vi "ParseRulesFile.vi"(8 "error in (no error)":errorcluster, 9 "Parameters":string, 11 "IRuleFileParser in":refnum<class "IRuleFileParser.lvclass">) -> (0 "error out":errorcluster, 2 "Rules":T1, 3 "IRuleFileParser out":refnum<class "IRuleFileParser.lvclass">)   [LabVIEW 2020, in "ExtensionInterfaces.lvlib" / "IRuleFileParser.lvclass"]
uses:
  IRuleFileParser.lvclass
  RulesDefinition.ctl
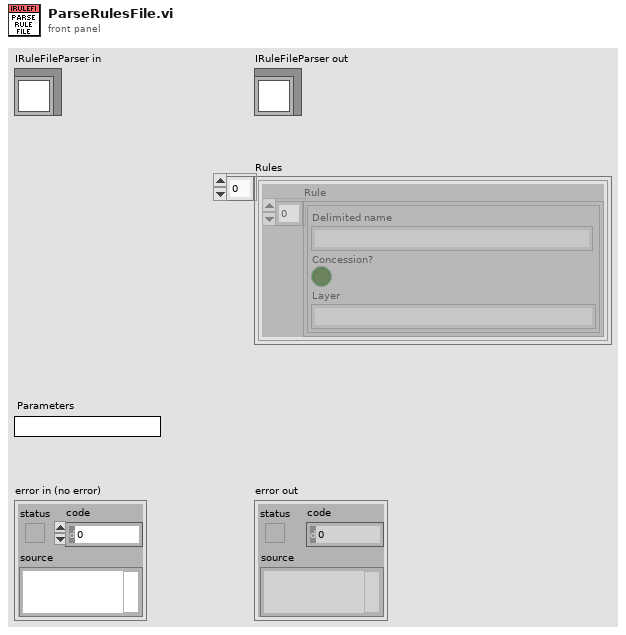
[diagram p1: front panel]
types:
  T1 = typedef "ExtensionInterfaces.lvlib/IRuleFileParser.lvclass/RulesDefinition.ctl" = cluster{"Rule":cluster{"Delimited name":string, "Concession?":bool, "Layer":string}[]}[]
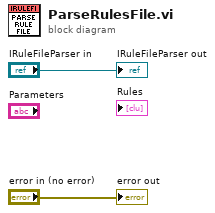
[diagram p0: block diagram]
diagram:
  "error out" <- "error in (no error)"
  "IRuleFileParser out" <- "IRuleFileParser in"
